vi "svx_Frequency Flat Chirp Pattern.vi"(10 "amplitude":dbl format="%.2f", 11 "samples":i32) -> (0 "error":i32, 3 "frequency flat chirp":dbl[](array[numeric]) format="%.2f")   [LabVIEW 2017]
uses:
  <vilib>/Analysis/2dsp.llb/Inverse Real FFT.vi
  <vilib>/Analysis/NI_AALPro.lvlib
  <vilib>/Analysis/NI_AALBase.lvlib
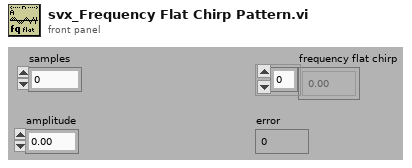
[diagram p1: front panel]
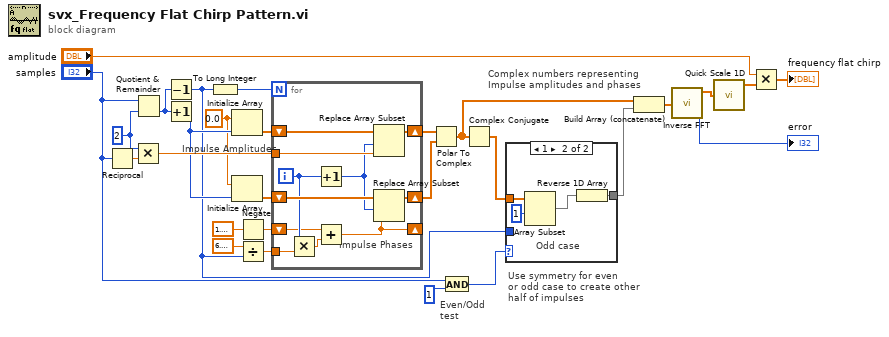
[diagram p0: block diagram]
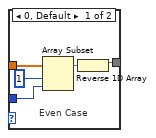
[diagram p2: hidden frame]
diagram:
  w8 = 0.0 ("Element Data")
  w11 = 2 ("y")
  # "Use symmetry for even\nor odd case to create other\nhalf of impulses"
  # "Even/Odd\ntest"
  # "Complex numbers representing \nImpulse amplitudes and phases"
  # "Impulse Amplitudes"
  n1 = Reciprocal(x="samples") -> (1/x=w16:dbl)
  n2 = Multiply(x=w11, y=w16) -> (x*y=w15:dbl)
  n3 = Quotient & Remainder(x="samples", y=w11) -> (floor(x/y)=w12:i32)  [unwired: 1 out]
  n4 = Decrement(x=w12) -> (x-1=w5:i32)
  n5 = Increment(x=w12) -> (x+1=w13:i32)
  n6 = To Long Integer(number=w5) -> (32bit integer=w14:i32)
  n7 = Initialize Array(w8, w13) -> (w27:dbl[])
  n8 = Initialize Array(w8, w13) -> (w26:dbl[])
  n9 = Negate(x=1.5707963267948966) -> (-x=w6:dbl)
  n10 = Divide(x=6.283185307179586, y=w5) -> (x/y=w9:dbl)
  n11 = for {
    N: w14 -> [_]
    tunnel: w15 -> [w39]
    shift-right: [w37] -> w24
    shift-left: w27 -> [w38]
    shift-right: [w36] -> w25
    shift-left: w26 -> [w35]
    tunnel: w9 -> [w32]
    shift-right: [w29] -> _
    shift-left: w6 -> [w30]
    i -> [w33]
    # "Impulse Phases"
    n12 = Multiply(x=w33, y=w32) -> (x*y=w31:dbl)
    n13 = Increment(x=w33) -> (x+1=w34:i32)
    n14 = Add(x=w30, y=w31) -> (x+y=w29:dbl)
    n15 = Replace Array Subset(array=w38, new element=w39, index=w34) -> (w37:dbl[])
    n16 = Replace Array Subset(array=w35, new element=w29, index=w34) -> (w36:dbl[])
  }
  n17 = Polar To Complex(1:w25, 2:w24) -> (0:w23:cdb[])
  n18 = And(x="samples", y=1 ("x")) -> (x .and. y?=w22:i32)
  n19 = Complex Conjugate(1:w23) -> (0:w21:cdb[])
  n20 = case shown="1" w22 {
    tunnel: [w44 w45] -> w19
    tunnel: w21 -> [w43 w48]
    tunnel: w5 -> [w40 _]
    frame 0, Default {
      # "Even Case"
      n21 = Array Subset(array=w43, index=1 ("Array Index"), length=w40) -> (w42:cdb[])
      n22 = Reverse 1D Array(array=w42) -> (reversed array=w44:cdb[])
    }
    frame 1 {
      # "Odd case"
      n23 = Array Subset(array=w48, index=1 ("Array Index")) -> (w46:cdb[])  [unwired: 1 in]
      n24 = Reverse 1D Array(array=w46) -> (reversed array=w45:cdb[])
    }
  }
  n25 = Build Array (concatenate)(w23, w19) -> (w20:cdb[])
  n26 = call-poly <vilib>:"Inverse FFT.vi"("FFT {X}"=w20) -> ("error"=→"error":i32, "X"=w17:dbl[])  [unwired: 9 in]
  n27 = call <vilib>:"Quick Scale 1D.vi"("X"=w17) -> ("Y[i]=X[i]/Max|X|"=w18:dbl[])  [unwired: 2 out]
  n28 = Multiply(x="amplitude", y=w18) -> (x*y=→"frequency flat chirp":dbl[])
